vi "Check Status.vi"(8 "error in (no error)":errorcluster, 11 "Power Supply in":refnum<class "Power Supply.lvclass">) -> (0 "error out":errorcluster, 1 "Status":string, 2 "Ready?":bool, 3 "Power Supply out":refnum<class "Power Supply.lvclass">)   [LabVIEW 2017, in "Power Supply.lvclass"]
uses:
  Power Supply.lvclass
  Power Supply.lvclass/Power Supply.ctl
  Global/Relative Sound Files.vi
panel:
  out "approach0?":bool
  out "Field":dbl[unit]
  out "Field sweep rate":dbl[unit]
  out "switchheater":bool caption="Switch Heater"
  out "persis?":bool caption="Persistent Mode"
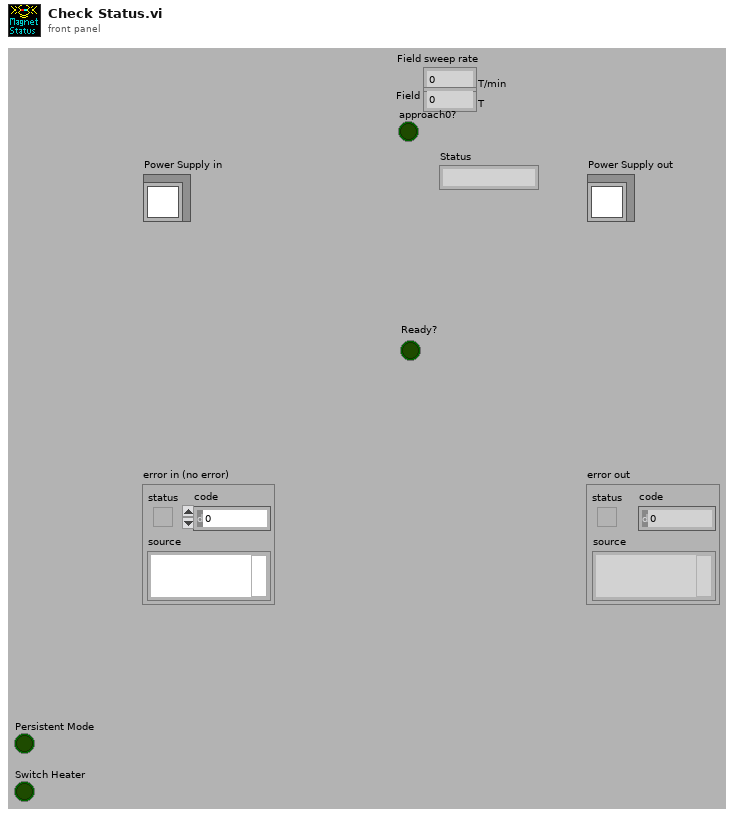
[diagram p1: front panel]
types:
  T1 = typedef "OxfordAddress.ctl" = cluster{"Com Port":i32, "ISOBUS Address":i32, "GPIB Address":i16, "Communication":enum16{"RS232", "ISOBUS", "GPIB", "Gateway"}}
  T2 = typedef "PSIO.ctl" = cluster{"Address":T1, "Version":enum16{"PS", "IPS"}}
  T3 = typedef "ILMRelayStatus.ctl" = cluster{"Shut down":bool, "Alarm sound":bool, "Alarm state":bool, "Silence prohib":bool, "Relay1 active":bool, "Relay 2 active":bool, "Relay 3 active":bool, "Relay 4 active":bool}
  T4 = cluster{"Value":i16, "At rest":bool, "Sweeping":bool, "Rate limiting":bool}
  T5 = cluster{"Value":i16, "Hold":bool, "To set point":bool, "To zero":bool, "Clamped":bool}
  T6 = cluster{"Value":i16, "Off (at zero field)":bool, "On":bool, "Off (at field)":bool, "No switch fitted":bool, "Confirm":bool}
  T7 = cluster{"Value":i16, "Quenched":bool, "Over heated":bool, "Warming up":bool}
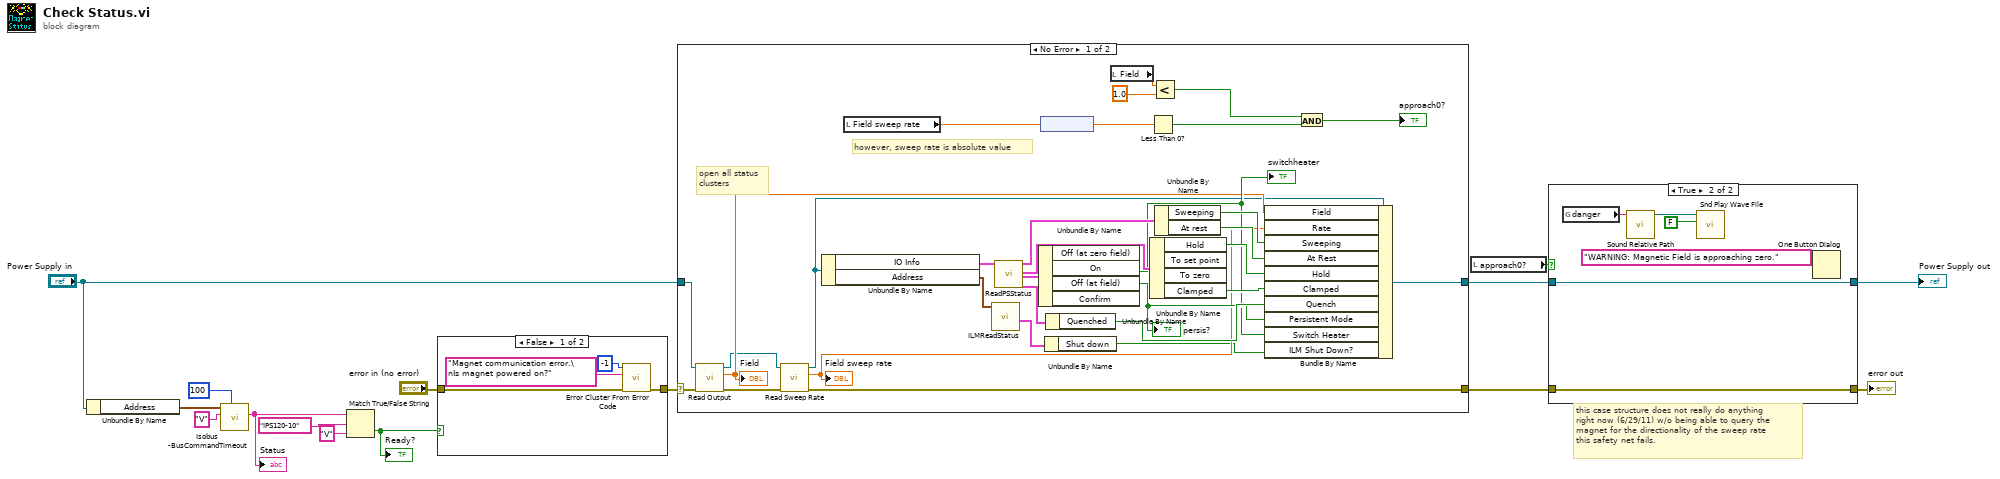
[diagram p0: block diagram]
diagram:
  # "this case structure does not really do anything\nright now (6/29/11) w/o being able to query the\nmagnet for the directionality of the sweep rate\nthis safety net fails."
  n1 = Unbundle By Name("Power Supply in") -> ("Address"=w11:T1)
  n2 = call "Isobus -BusCommandTimeout.vi"("Timeout (ms)"=100, "Command"="V", "Address"=w11) -> ("Reply"=w15:string)  [unwired: 5 out]
  "Status" <- w15
  n3 = Match True/False String(2:"V", 3:"IPS120-10", 4:w15) -> (0:w6:bool)  [unwired: 1 out]
  "Ready?" <- w6
  n4 = case shown="False" w6 {
    tunnel: "error in (no error)" -> [w17 w20]
    tunnel: [w16 w20] -> w7
    frame False {
      n5 = call <vilib>:"Error Cluster From Error Code.vi"("error in (no error)"=w17, "error message (\"\")"="Magnet communication error.\nIs magnet powered on?" ("error message (\"\")"), "error code (0)"=-1) -> ("error out"=w16:errorcluster)  [unwired: 6 in]
    }
    frame True {
    }
  }
  n6 = case shown="No Error" w7 {
    selector: w7 -> [w34 w52]
    tunnel: "Power Supply in" -> [w37 w53]
    tunnel: [w38 w53] -> w5
    tunnel: [w33 w52] -> w4
    frame No Error {
      # "however, sweep rate is absolute value"
      # "open all status\nclusters"
      n7 = call-dynamic "Read Output.vi"("error in (no error)"=w34, "Power Supply in"=w37) -> ("error out"=w35:errorcluster, "Field"=w40:dbl[unit], "Power Supply out"=w36:refnum<class "Power Supply.lvclass">)  [unwired: 5 in, 2 out]
      "Field" <- w40
      n8 = call-dynamic "Read Sweep Rate.vi"("error in (no error)"=w35, "Power Supply in"=w36) -> ("error out"=w33:errorcluster, "Field sweep rate"=w39:dbl[unit], "Power Supply out"=w32:refnum<class "Power Supply.lvclass">)  [unwired: 7 in]
      "Field sweep rate" <- w39
      n9 = Unbundle By Name(w32) -> ("IO Info"=w31:T2, "Address"=w23:T1)
      n10 = local read "Field sweep rate"() -> (w28:dbl[unit])
      n11 = call "ILMReadStatus.vi"("Instrument address"=w23) -> ("Relay"=w22:T3)  [unwired: 3 in, 3 out]
      n12 = call "ReadPSStatus.vi"("IO Info"=w31) -> ("Mode (n)"=w49:T4, "Activity"=w51:T5, "Switch Heater"=w50:T6, "System Status (m)"=w48:T7)  [unwired: 15 out]
      n13 = Unbundle By Name(w50) -> ("On"=w41:bool, "Off (at field)"=w42:bool)  [unwired: 2 out]
      "persis?" <- w42
      "switchheater" <- w41
      n14 = node(w28) -> (w27:dbl)
      n15 = Unbundle By Name(w22) -> ("Shut down"=w21:bool)
      n16 = Unbundle By Name(w48) -> ("Quenched"=w45:bool)
      n17 = local read "Field"() -> (w25:dbl[unit])
      n18 = Less Than 0?(x=w27) -> (x < 0?=w29:bool)
      n19 = Unbundle By Name(w51) -> ("Hold"=w43:bool, "Clamped"=w46:bool)  [unwired: 2 out]
      n20 = Less?(x=w25, y=dbl[unit] 1.0) -> (x < y?=w30:bool)
      n21 = Unbundle By Name(w49) -> ("Sweeping"=w47:bool, "At rest"=w44:bool)
      n22 = Bundle By Name(cluster=w32, "Field"=w40, "Rate"=w39, "Sweeping"=w47, "At Rest"=w44, "Hold"=w43, "Clamped"=w46, "Quench"=w45, "Persistent Mode"=w42, "Switch Heater"=w41, "ILM Shut Down?"=w21) -> (w38:refnum<class "Power Supply.lvclass">)
      n23 = And(x=w30, y=w29) -> (x .and. y?=→"approach0?":bool)
    }
    frame Error {
    }
  }
  n24 = local read "approach0?"() -> (w1:bool)
  n25 = case shown="True" w1 {
    tunnel: w5 -> [w55 w57]
    tunnel: w4 -> [w54 w58]
    tunnel: [w54 w58] -> w3
    tunnel: [w55 w57] -> w2
    frame False {
    }
    frame True {
      n26 = global read "Relative Sound Files.vi" "danger"() -> (w60:string)
      n27 = call "Sound Relative Path.vi"("Sound"=w60) -> ("Relative Path"=w59:path)  [unwired: 10 in]
      n28 = call <vilib>:"Snd Play Wave File.vi"("wait until finish (T)"=FALSE, "wave file path"=w59) -> ()  [unwired: 1 in, 9 out]
      n29 = One Button Dialog(message="WARNING: Magnetic Field is approaching zero.") -> ()  [unwired: 1 in, 1 out]
    }
  }
  "Power Supply out" <- w2
  "error out" <- w3
